vi "SendToDeleteRecord.vi"(8 "error in (no error)":errorcluster, 9 "message value":variant) -> (0 "error out":errorcluster)   [LabVIEW 2015, in "FileHandler.lvlib"]
uses:
  FileHandler.lvlib
  <vilib>/addons/Qbus/Qbus.lvclass
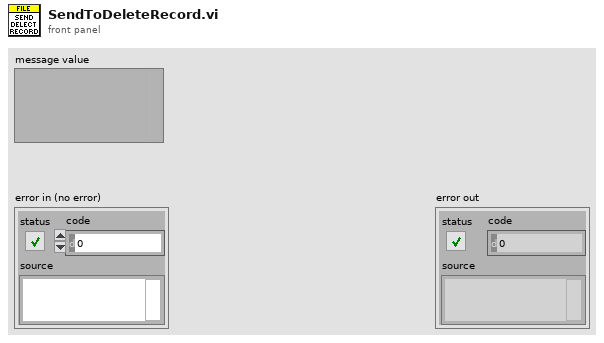
[diagram p1: front panel]
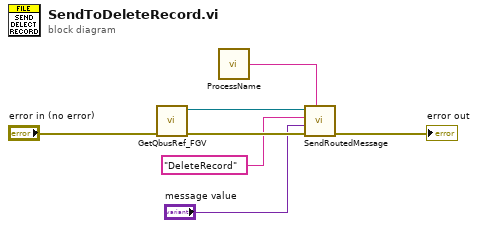
[diagram p0: block diagram]
diagram:
  n1 = call <vilib>:"GetQbusRef_FGV.vi"("error in (no error)"="error in (no error)") -> ("error out"=w6:errorcluster, "Qbus out"=w7:refnum<class "Qbus.lvclass">)  [unwired: 9 in]
  n2 = call "ProcessName.vi"() -> ("process name"=w5:string)  [unwired: 5 in]
  n3 = call <vilib>:"SendRoutedMessage.vi"("listener process"=w5, "error in (no error)"=w6, "message value"="message value", "message name"="DeleteRecord", "Qbus in"=w7) -> ("error in (no error)"=→"error out":errorcluster)  [unwired: 5 in, 1 out]
